vi "Set Initialization Data - Aging View.vi"(8 "error in":errorcluster, 11 "Main View in":refnum<class "Main View.lvclass">) -> (0 "error out":errorcluster, 3 "Main View out":refnum<class "Main View.lvclass">)   [LabVIEW 2018, in "Main View.lvclass"]
doc: "Sets the initialization data of a statically linked subWorker."
uses:
  Main View.lvclass
  Aging View/Initialization Data.ctl
  <vilib>/addons/_Workers/Library/Classes/Message Queue/Message Queue.lvclass
  Main View.lvclass/Main View.ctl
  <vilib>/addons/_Workers/Library/Classes/Worker/Worker.lvclass/Worker.ctl
  Acquire Data/Acquire Data.lvclass
  D:/Program Files (x86)/National Instruments/LabVIEW 2018/vi.lib/addons/_Workers/Library/Classes/Worker/Worker.lvclass
  Aging View/Aging View.lvclass
  <vilib>/addons/_Workers/Library/Classes/Worker/Worker.lvclass
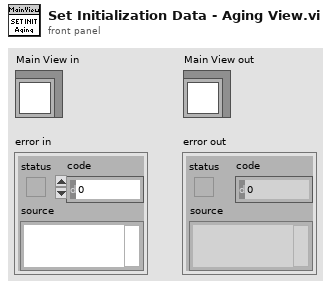
[diagram p1: front panel]
types:
  T1 = typedef "Aging View.lvclass/Initialization Data.ctl" = cluster{"MainPanel":refnum<vi>, "Acquire Queue":refnum<class "Message Queue.lvclass">}
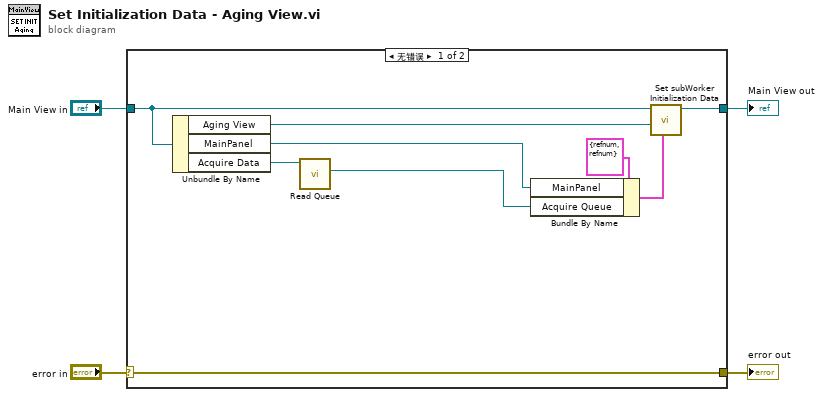
[diagram p0: block diagram]
diagram:
  n1 = case shown="无错误" "error in" {
    selector: "error in" -> [w13 w15]
    tunnel: [w13 w15] -> w3
    tunnel: [w11 w14] -> w2
    tunnel: "Main View in" -> [w10 w14]
    frame No Error {
      n2 = Unbundle By Name(w10) -> ("Aging View"=w12:refnum<class "Aging View.lvclass">, "MainPanel"=w7:refnum<vi>, "Acquire Data"=w6:refnum<class "Acquire Data.lvclass">)
      n3 = call <vilib>:"Read Queue.vi"("Worker"=w6) -> ("Message Queue out"=w5:refnum<class "Message Queue.lvclass">)  [unwired: 9 in, 1 out]
      n4 = Bundle By Name(cluster=T1 {"MainPanel"=refnum, "Acquire Queue"=refnum} ("Initialization Data"), "MainPanel"=w7, "Acquire Queue"=w5) -> (w8:T1)
      n5 = call-dynamic "Set subWorker Initialization Data.vi"("Initialization Data"=w8, "subWorker"=w12, "Worker"=w10) -> ("Worker out"=w11:refnum<class "Main View.lvclass">)  [unwired: 8 in]
    }
    frame Error {
    }
  }
  "error out" <- w3
  "Main View out" <- w2
